vi "pztCtrl.vi"() -> ()   [LabVIEW 2017]
uses:
  <vilib>/DAQmx/write.llb/DAQmx Write (Analog 2D DBL NChan NSamp).vi
  <vilib>/DAQmx/create/channels.llb/DAQmx Create Channel (AO-Voltage-Basic).vi
  <vilib>/DAQmx/configure/timing.llb/DAQmx Timing (Sample Clock).vi
  <vilib>/DAQmx/miscellaneous.llb/DAQmx Fill In Error Info.vi
panel:
  in  "stop":bool
  out "Consistancy2":dbl
  out "Consistancy1":dbl
  in  "DutyLength2":dbl=0.2
  in  "DutyLength1":dbl=0.2
  in  "WaveParameters2":T1={"Amplitude"=1.0, "Frequency"=0, "PhaseOffset"=0.0}
  in  "FolderParameters2":T2={"FolderShape"=enum."Linear", "FolderInitial"=1.0, "FolderFinal"=1.0}
  in  "WaveParameters1":T1={"Amplitude"=1.0, "Frequency"=0, "PhaseOffset"=0.0}
  in  "FolderParameters1":T2={"FolderShape"=enum."Linear", "FolderInitial"=1.0, "FolderFinal"=1.0}
  in  "Angle2":dbl
  in  "Angle1":dbl
  in  "WaveParameters2":T1={"Amplitude"=1.0, "Frequency"=0, "PhaseOffset"=0.0}
  in  "FolderParameters2":T2={"FolderShape"=enum."Linear", "FolderInitial"=1.0, "FolderFinal"=1.0}
  in  "WaveParameters1":T1={"Amplitude"=1.0, "Frequency"=0, "PhaseOffset"=0.0}
  in  "FolderParameters1":T2={"FolderShape"=enum."Linear", "FolderInitial"=1.0, "FolderFinal"=1.0}
  in  "Start":bool
  out "V2":dbl[](graph)
  out "V1":dbl[](graph)
  in  "DAQmx Device Name":tag="Dev1"
  in  "Duty Length":dbl=0.5
  in  "Sampling Rate":i32=1000000
  in  "fps":dbl=10.0
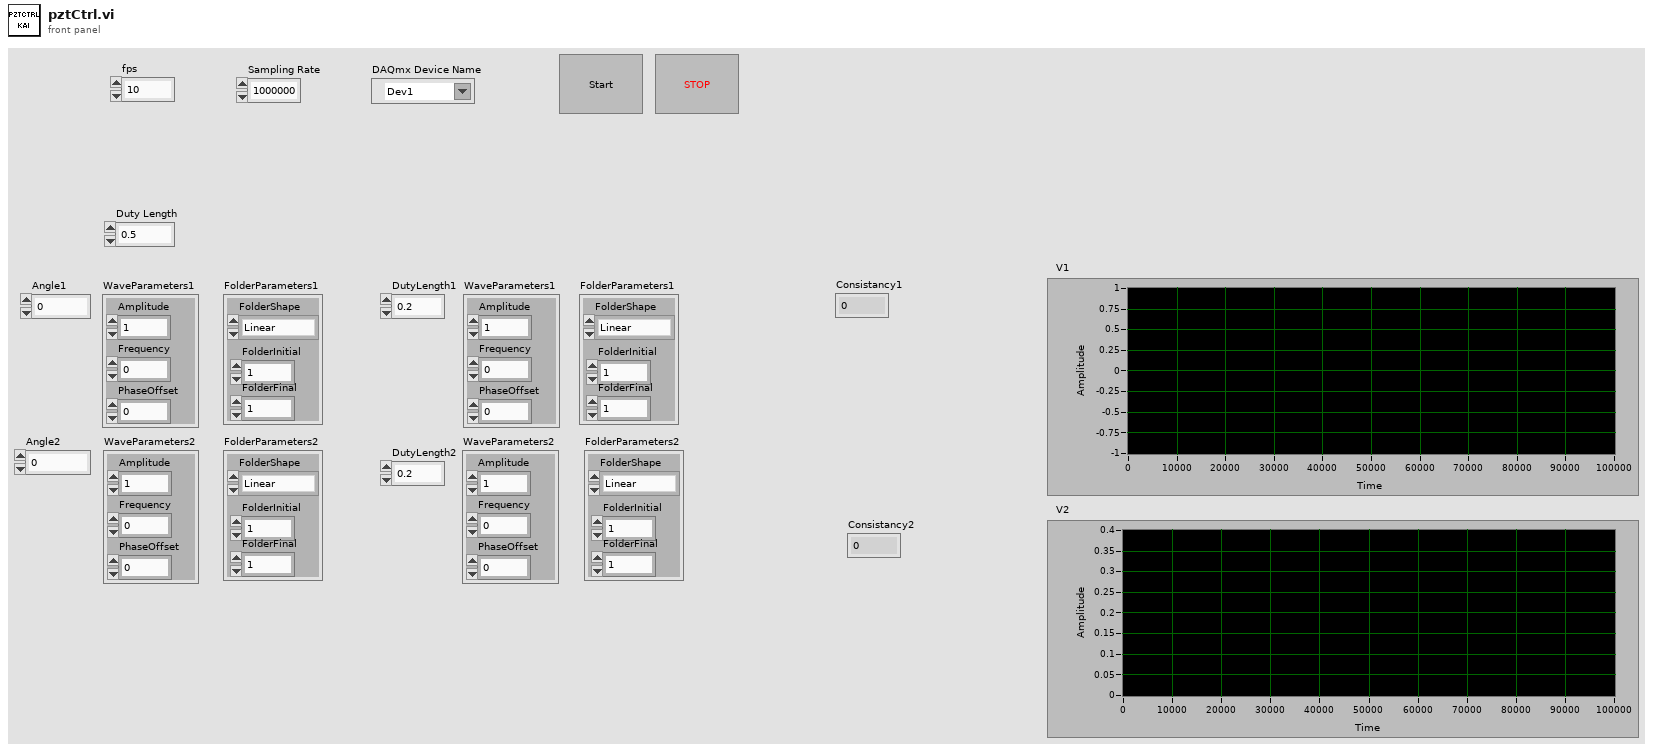
[diagram p1: front panel]
types:
  T1 = cluster{"Amplitude":dbl, "Frequency":i32, "PhaseOffset":dbl}
  T2 = cluster{"FolderShape":enum16{"Linear", "Exponential"}, "FolderInitial":dbl, "FolderFinal":dbl}
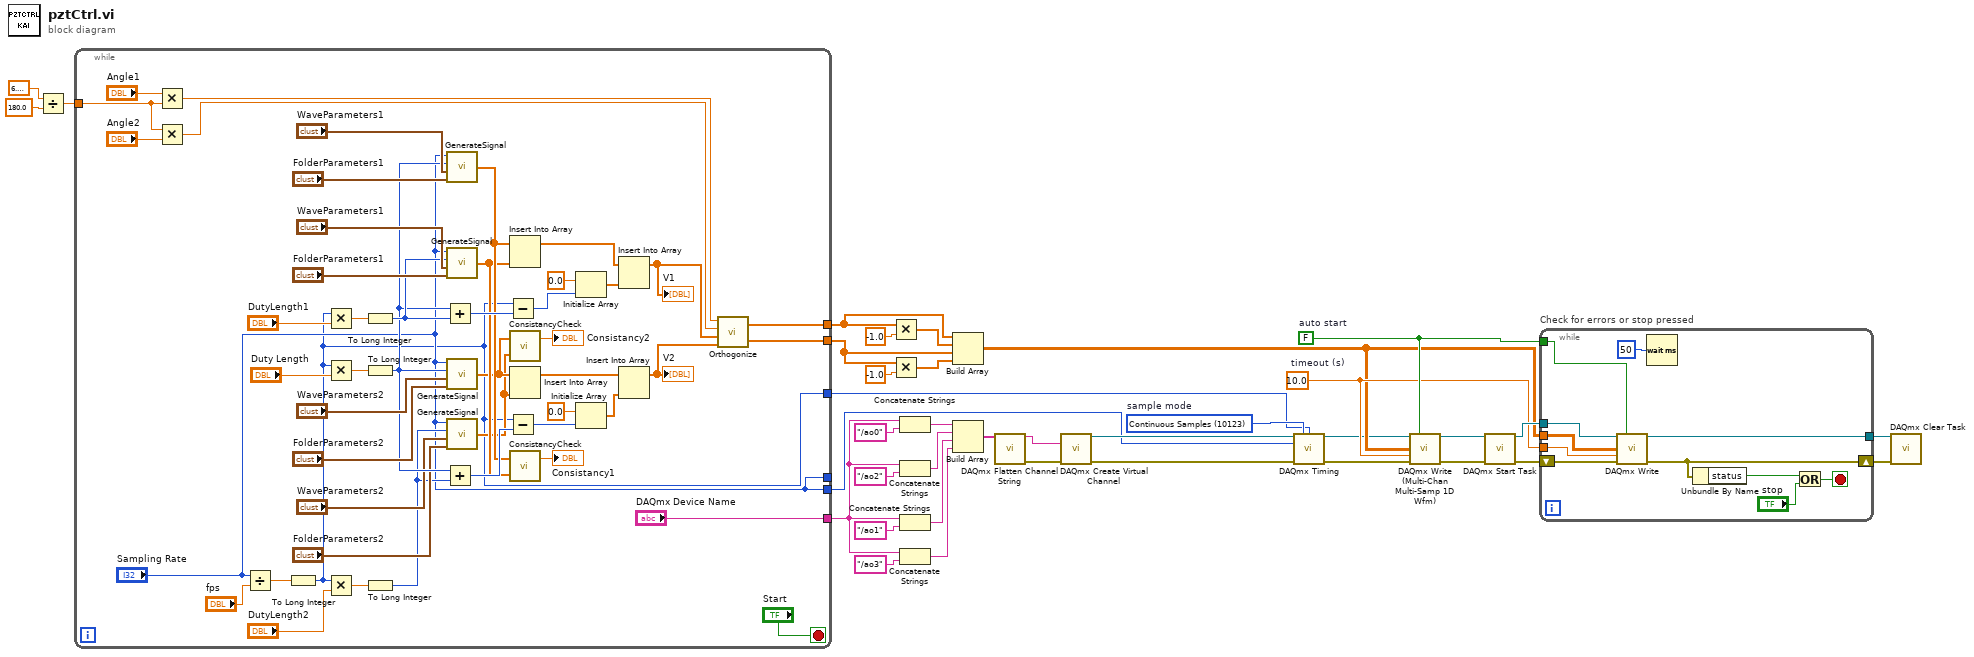
[diagram p0: block diagram]
diagram:
  w14 = 10123 items=["Finite Samples"=10178, "Continuous Samples"=10123, "Hardware Timed Single Point"=12522]  # sample mode
  w16 = 10.0  # timeout (s)
  w17 = FALSE  # auto start
  n1 = Divide(x=6.283185307179586, y=180.0) -> (x/y=w28:dbl)
  n2 = while {
    tunnel: ["Sampling Rate"] -> _
    tunnel: ["DAQmx Device Name"] -> w24
    tunnel: w28 -> [w49]
    tunnel: [w47] -> w26
    tunnel: [w46] -> w27
    tunnel: ["Sampling Rate"] -> w2
    tunnel: [w38] -> w1
    stop <- "Start" stop-if-true
    n3 = Multiply(x="Angle1", y=w49) -> (x*y=w51:dbl)
    n4 = Multiply(x=w49, y="Angle2") -> (x*y=w52:dbl)
    n5 = Divide(x="Sampling Rate", y="fps") -> (x/y=w77:dbl)
    n6 = To Long Integer(number=w77) -> (32bit integer=w38:i32)
    n7 = Multiply(x=w38, y="DutyLength1") -> (x*y=w79:dbl)
    n8 = Multiply(x=w38, y="Duty Length") -> (x*y=w83:dbl)
    n9 = Multiply(x=w38, y="DutyLength2") -> (x*y=w78:dbl)
    n10 = To Long Integer(number=w79) -> (32bit integer=w59:i32)
    n11 = To Long Integer(number=w83) -> (32bit integer=w56:i32)
    n12 = To Long Integer(number=w78) -> (32bit integer=w53:i32)
    n13 = Add(x=w56, y=w59) -> (x+y=w74:i32)
    n14 = Add(x=w56, y=w53) -> (x+y=w68:i32)
    n15 = call "GenerateSignal.vi"("FolderParameters"="FolderParameters1", "WaveParameters"="WaveParameters1", "Number of Samples"=w56, "Sampling Rate"="Sampling Rate") -> ("Wave"=w45:dbl[])
    n16 = call "GenerateSignal.vi"("FolderParameters"="FolderParameters1", "WaveParameters"="WaveParameters1", "Number of Samples"=w59, "Sampling Rate"="Sampling Rate") -> ("Wave"=w44:dbl[])
    n17 = call "GenerateSignal.vi"("FolderParameters"="FolderParameters2", "WaveParameters"="WaveParameters2", "Number of Samples"=w56, "Sampling Rate"="Sampling Rate") -> ("Wave"=w43:dbl[])
    n18 = call "GenerateSignal.vi"("FolderParameters"="FolderParameters2", "WaveParameters"="WaveParameters2", "Number of Samples"=w53, "Sampling Rate"="Sampling Rate") -> ("Wave"=w42:dbl[])
    n19 = Subtract(x=w38, y=w74) -> (x-y=w76:i32)
    n20 = Subtract(x=w38, y=w68) -> (x-y=w71:i32)
    n21 = Insert Into Array(array=w45, new element=w44) -> (w73:dbl[])  [unwired: 1 in]
    n22 = call "ConsistancyCheck.vi"("Input 2"=w42, "Input 1"=w43) -> ("Difference"=→"Consistancy2":dbl)  [unwired: 1 out]
    n23 = Insert Into Array(array=w43, new element=w42) -> (w67:dbl[])  [unwired: 1 in]
    n24 = call "ConsistancyCheck.vi"("Input 2"=w44, "Input 1"=w45) -> ("Difference"=→"Consistancy1":dbl)  [unwired: 1 out]
    n25 = Initialize Array(0.0 ("element"), w76) -> (w72:dbl[])
    n26 = Initialize Array(0.0 ("element"), w71) -> (w69:dbl[])
    n27 = Insert Into Array(array=w73, new element=w72) -> (w65:dbl[])  [unwired: 1 in]
    "V1" <- w65
    n28 = Insert Into Array(array=w67, new element=w69) -> (w66:dbl[])  [unwired: 1 in]
    "V2" <- w66
    n29 = call "Orthogonize.vi"("b"=w66, "a"=w65, "Theta2"=w52, "Theta1"=w51) -> ("y"=w47:dbl[], "x"=w46:dbl[])
  }
  n30 = Multiply(x=w27, y=-1.0) -> (x*y=w35:dbl[])
  n31 = Multiply(x=w26, y=-1.0) -> (x*y=w25:dbl[])
  n32 = Concatenate Strings(w24, "/ao0" ("string")) -> (w11:string)
  n33 = Concatenate Strings(w24, "/ao2" ("string")) -> (w10:string)
  n34 = Concatenate Strings(w24, "/ao1" ("string")) -> (w9:string)
  n35 = Concatenate Strings(w24, "/ao3" ("string")) -> (w8:string)
  n36 = Build Array(w27, w35, w26, w25) -> (w15:dbl[][])
  n37 = Build Array(w11, w10, w9, w8) -> (w7:string[])
  n38 = call <vilib>:"DAQmx Flatten Channel String.vi"("names in"=w7) -> ("names out"=w6:string, "error out"=w3:errorcluster)  [unwired: 13 in]
  n39 = call-poly <vilib>:"DAQmx Create Virtual Channel.vi"("physical channels"=w6, "error in"=w3) -> ("task out"=w5:refnum<k21>, "error out"=w4:errorcluster)  [unwired: 12 in]
  n40 = call-poly <vilib>:"DAQmx Timing.vi"("task/channels in"=w5, "sample mode"=w14, "samples per channel"=w1, "rate"=w2, "error in"=w4) -> ("task out"=w13:refnum<k21>, "error out"=w12:errorcluster)  [unwired: 9 in]
  n41 = call-poly "DAQmx Write (Multi-Chan Multi-Samp 1D Wfm).vi"("task/channels in"=w13, "auto start"=w17, "data"=w15, "timeout"=w16, "error in"=w12) -> ("task out"=w20:refnum<k21>, "error out"=w19:errorcluster)  [unwired: 8 in, 1 out]
  n42 = call <vilib>:"DAQmx Start Task.vi"("task/channels in"=w20, "error in"=w19) -> ("task out"=w22:refnum<k21>, "error out"=w23:errorcluster)  [unwired: 12 in]
  n43 = while "Check for errors or stop pressed" {
    tunnel: [w93] -> w18
    tunnel: w22 -> [w94]
    shift-right: [w90] -> w21
    shift-left: w23 -> [w92]
    tunnel: w17 -> [w88]
    tunnel: w16 -> [w87]
    tunnel: w15 -> [w86]
    stop <- w95 stop-if-true
    n44 = call-poly <vilib>:"DAQmx Write.vi"("task/channels in"=w94, "auto start"=w88, "data"=w86, "timeout"=w87, "error in"=w92) -> ("task out"=w93:refnum<k21>, "error out"=w90:errorcluster)  [unwired: 8 in, 1 out]
    n45 = Wait (ms)(milliseconds to wait=u32 50) -> ()  [unwired: 1 out]
    n46 = Unbundle By Name(w90) -> ("status"=w91:bool)
    n47 = Or(x=w91, y="stop") -> (x .or. y?=w95:bool)
  }
  n48 = call <vilib>:"DAQmx Clear Task.vi"("task in"=w18, "error in"=w21) -> ()  [unwired: 13 in, 1 out]
